vi "CloseRunningVIs.vi"(8 "error in (no error)":errorcluster, 10 "VI name":string, 11 "Target":string) -> (0 "error out":errorcluster)   [LabVIEW 2011]
doc: "Closes the chosen VI on the selected target if it is running.\n\n\nVersion 1.0 - 10/21/2009\n\nPhaeron, Inc.\nwww.phaeron.com\ninfo@phaeron.com"
panel:
  out "Matches":i32[](array[numeric])
  out "App.AllVIs":string[](array[string])
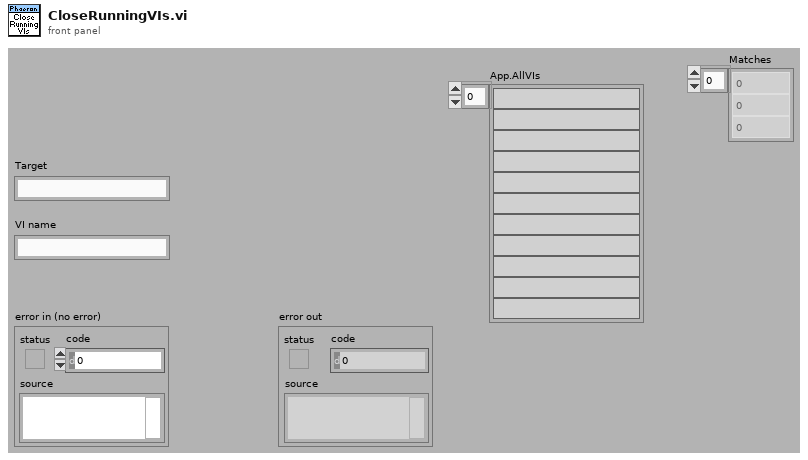
[diagram p1: front panel]
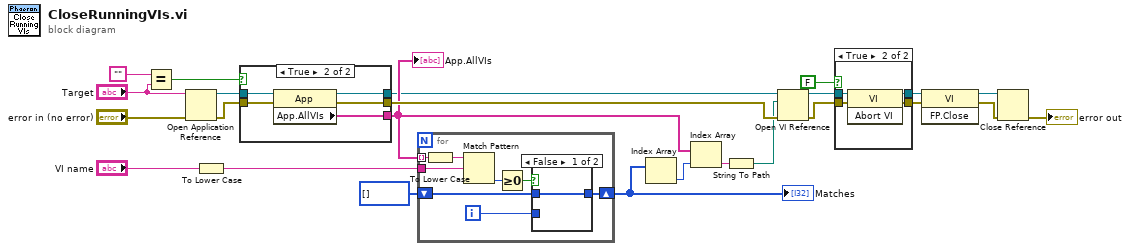
[diagram p0: block diagram]
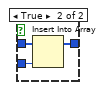
[diagram p3: hidden frame]
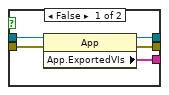
[diagram p4: hidden frame]
diagram:
  n1 = Equal?(x="", y="Target") -> (x = y?=w20:bool)
  n2 = Open Application Reference(8:"error in (no error)", 11:"Target") -> (0:w23:errorcluster, 3:w24:refnum<vi>)  [unwired: 2 in]
  n3 = To Lower Case(string="VI name") -> (all lower case string=w17:string)
  n4 = case shown="True" w20 {
    tunnel: w24 -> [w29 w34]
    tunnel: w23 -> [w28 w33]
    tunnel: [w27 w32] -> w8
    tunnel: [w26 w31] -> w16
    tunnel: [w25 w30] -> w3
    frame False {
      n5 = property class="App"(reference=w29, error in=w28) -> (reference out=w25:refnum<vi>, error out=w26:errorcluster, "App.ExportedVIs"=w27:string[])
    }
    frame True {
      n6 = property class="App"(reference=w34, error in=w33) -> (reference out=w30:refnum<vi>, error out=w31:errorcluster, "App.AllVIs"=w32:string[])
    }
  }
  "App.AllVIs" <- w8
  n7 = for {
    tunnel: w8 -> [w42] mode=indexing
    tunnel: w17 -> [w41]
    shift-right: [w38] -> w10
    shift-left: i32[] [] -> [w37]
    i -> [w36]
    n8 = To Lower Case(string=w42) -> (all lower case string=w35:string)
    n9 = Match Pattern(string=w35, regular expression=w41) -> (offset past match=w40:i32)  [unwired: 1 in, 3 out]
    n10 = Greater Or Equal To 0?(x=w40) -> (x >= 0?=w39:bool)
    n11 = case shown="False" w39 {
      tunnel: [w43 w44] -> w38
      tunnel: w37 -> [w43 w46]
      tunnel: w36 -> [_ w45]
      frame False {
      }
      frame True {
        n12 = Insert Into Array(array=w46, new element=w45) -> (w44:i32[])  [unwired: 1 in]
      }
    }
  }
  "Matches" <- w10
  n13 = Index Array(array=w10) -> (element=w9:i32)  [unwired: 1 in]
  n14 = Index Array(array=w8, index=w9) -> (element=w7:string)
  n15 = String To Path(string=w7) -> (path=w6:path)
  n16 = Open VI Reference(application reference (local)=w3, vi path=w6, error in (no error)=w16) -> (vi reference=w15:refnum<vi>, error out=w11:errorcluster)  [unwired: 3 in]
  n17 = case shown="True" FALSE {
    tunnel: w15 -> [w48 w52]
    tunnel: [w48 w51] -> w14
    tunnel: [w47 w50] -> w13
    tunnel: w11 -> [w47 w49]
    frame False {
    }
    frame True {
      n18 = invoke class="VI" method="Abort VI"(reference=w52, error in=w49) -> (reference out=w51:refnum<vi>, error out=w50:errorcluster)  [unwired: 1 in, 1 out]
    }
  }
  n19 = invoke class="VI" method="FP.Close"(reference=w14, error in=w13) -> (reference out=w4:refnum<vi>, error out=w12:errorcluster)  [unwired: 1 in, 1 out]
  n20 = Close Reference(reference=w4, error in (no error)=w12) -> (error out=→"error out":errorcluster)
